vi "VisaRWGen.vi"(0 "VISA Rsrc":refnum<visa-resource-name>="SR530", 1 "2Lecture?":bool, 2 "EOS (Aucun)":string, 3 "ReadDelay (0 ms)":u32, 5 "ChaineCom":string caption="Chaîne de commande", 9 "Nbcaract":u32=100 caption="Nombre de \ncaractères à lire", 11 "error in (no error)":errorcluster, 12 "Lecture?(T)":bool=TRUE, 13 "Timeout ms":u32=1000) -> (4 "VISA Rsrc Out":refnum<visa-resource-name>="GPIB0::12::INSTR", 6 "ChaineRep":string caption="Chaîne de réponse", 8 "ChaineRep2":string caption="Chaîne de réponse 2", 10 "Count out 2":u32=44 caption="Nombre de caractères lus 2", 14 "Count out":u32=44 caption="Nombre de caractères lus", 15 "error out":errorcluster)   [LabVIEW 2019]
doc: "Ce VI envoie des commande d'écriture et de lecture VISA à l'appareil GPIB. Il permet de ne pas séparer un question de sa réponse. Pour que cela fonctionne toute lecture d'un instrument doit se faire par ce VI."
panel:
  in  "Write?(T)":bool=TRUE
  in  "ClosePort":bool
  out "Sent Byte 0":u8
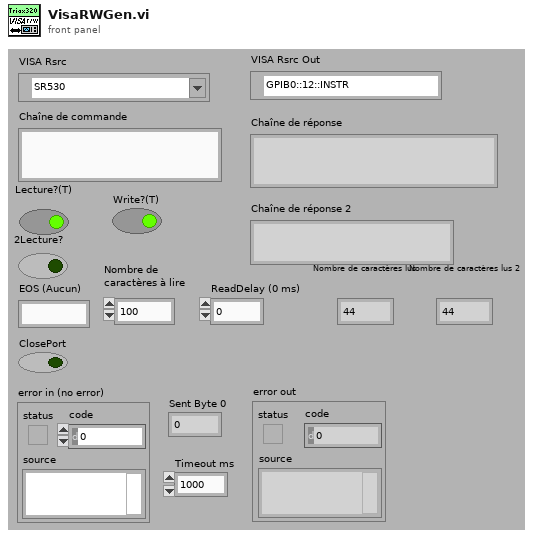
[diagram p1: front panel]
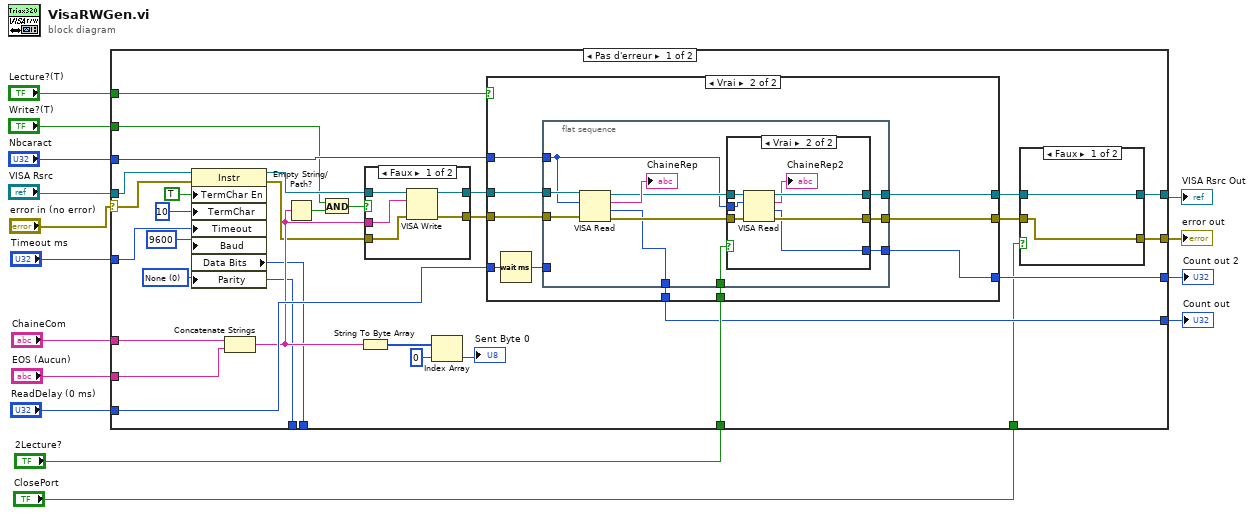
[diagram p0: block diagram]
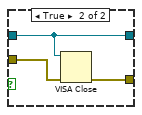
[diagram p2: hidden frame]
diagram:
  n1 = case shown="Pas d'erreur" "error in (no error)" {
    selector: "error in (no error)" -> [w31 w93]
    tunnel: "VISA Rsrc" -> [w33 w92]
    tunnel: [w20 w92] -> w7
    tunnel: "ChaineCom" -> [w47 _]
    tunnel: "EOS (Aucun)" -> [w24 _]
    tunnel: "ReadDelay (0 ms)" -> [w44 _]
    tunnel: "Nbcaract" -> [w43 _]
    tunnel: "Lecture?(T)" -> [w42 _]
    tunnel: [w22 w93] -> w9
    tunnel: "2Lecture?" -> [w41 _]
    tunnel: [w36 _] -> w5
    tunnel: [w35 _] -> w4
    tunnel: "Timeout ms" -> [w28 _]
    tunnel: [w27 _] -> _
    tunnel: [w25 _] -> _
    tunnel: "ClosePort" -> [w19 _]
    tunnel: "Write?(T)" -> [w16 _]
    frame No Error {
      w25 = u16 0 items=["None", "Odd", "Even", "Mark", "Space"] ("Serial Settings:Parity")
      n2 = property class="Instr"(reference=w33, error in=w31, "TermChar En"=TRUE ("Message Based Settings:Termination Character Enable"), "TermChar"=u8 10 ("Message Based Settings:Termination Character"), "Timeout"=w28, "Baud"=u32 9600 ("Serial Settings:Baud Rate"), "Parity"=w25) -> (reference out=w34:refnum<visa-resource-name>, error out=w32:errorcluster, "Data Bits"=w27:u16)
      n3 = Concatenate Strings(w47, w24) -> (w37:string)
      n4 = Empty String/Path?(string/path=w37) -> (empty?=w17:bool)
      n5 = And(x=w16, y=w17) -> (x .and. y?=w18:bool)
      n6 = String To Byte Array(string=w37) -> (unsigned byte array=w40:u8[])
      n7 = case shown="Faux" w18 {
        tunnel: w34 -> [w57 w59]
        tunnel: w32 -> [w53 w58]
        tunnel: [w56 w59] -> w46
        tunnel: [w55 w58] -> w45
        tunnel: w37 -> [w54 _]
        frame False {
          n8 = VISA Write(VISA resource name=w57, write buffer=w54, error in (no error)=w53) -> (VISA resource name out=w56:refnum<visa-resource-name>, error out=w55:errorcluster)  [unwired: 1 out]
        }
        frame True {
        }
      }
      n9 = Index Array(array=w40, index=0 ("indice")) -> (element=→"Sent Byte 0":u8)
      n10 = case shown="Vrai" w42 {
        tunnel: w46 -> [w61 w71]
        tunnel: [w61 w70] -> w21
        tunnel: w45 -> [w60 w69]
        tunnel: [w60 w68] -> w23
        tunnel: w43 -> [_ w67]
        tunnel: w44 -> [_ w66]
        tunnel: w41 -> [_ w64]
        tunnel: [_ w63] -> w36
        tunnel: [_ w62] -> w35
        frame False {
        }
        frame True {
          n11 = Wait (ms)(milliseconds to wait=w66) -> (millisecond timer value=w65:u32)
          n12 = flat-sequence {
            tunnel: [w78] -> w68
            tunnel: [w76] -> w70
            tunnel: w71 -> [w82]
            tunnel: w69 -> [w80]
            tunnel: w67 -> [w74]
            tunnel: w65 -> [_]
            tunnel: w64 -> [w75]
            tunnel: [w73] -> w63
            tunnel: [w72] -> w62
            frame #0 {
              n13 = VISA Read(VISA resource name=w82, byte count=w74, error in (no error)=w80) -> (VISA resource name out=w77:refnum<visa-resource-name>, read buffer=→"ChaineRep":string, return count=w72:u32, error out=w79:errorcluster)
              n14 = case shown="Vrai" w75 {
                tunnel: w79 -> [w83 w91]
                tunnel: [w83 w90] -> w78
                tunnel: w77 -> [w84 w89]
                tunnel: [w84 w88] -> w76
                tunnel: w74 -> [_ w86]
                tunnel: [_ w85] -> w73
                frame False {
                }
                frame True {
                  n15 = VISA Read(VISA resource name=w89, byte count=w86, error in (no error)=w91) -> (VISA resource name out=w88:refnum<visa-resource-name>, read buffer=→"ChaineRep2":string, return count=w85:u32, error out=w90:errorcluster)
                }
              }
            }
          }
        }
      }
      n16 = case shown="Faux" w19 {
        tunnel: w23 -> [w49 w52]
        tunnel: [w49 w51] -> w22
        tunnel: w21 -> [w48 w50]
        tunnel: [w48 w50] -> w20
        frame False {
        }
        frame True {
          n17 = VISA Close(VISA resource name=w50, error in (no error)=w52) -> (error out=w51:errorcluster)
        }
      }
    }
    frame Error {
    }
  }
  "error out" <- w9
  "VISA Rsrc Out" <- w7
  "Count out 2" <- w5
  "Count out" <- w4
